vi "NI-USB6212.vi"() -> ()   [LabVIEW 2020]
uses:
  <vilib>/Utility/miscctls.llb/LVPointTypeDef.ctl
  LabVIEW 2020 Toolkits/toolkits_lv2020_32bit/Synchronization.llb/SynchRefs_SetGet.ctl
  LabVIEW 2020 Toolkits/VI Server Toolkit/VI Server Libraries/VI Server_GetControl.llb/VI Server_STR_Get.vi
  LabVIEW 2020 Toolkits/VI Server Toolkit/VI Server Libraries/VI Server_Set Controls.llb/Set STR Control.vi
  LabVIEW 2020 Toolkits/VI Server Toolkit/VI Server Libraries/VI Server_GetControl.llb/VI Server_DBL_Get.vi
  LabVIEW 2020 Toolkits/VI Server Toolkit/VI Server Libraries/VI Server_GetControl.llb/VI Server_Slide_DBL_Get.vi
  LabVIEW 2020 Toolkits/VI Server Toolkit/VI Server Libraries/VI Server_GetControl.llb/VI Server_DAQmx_Device_Get.vi
  LabVIEW 2020 Toolkits/VI Server Toolkit/VI Server Toolkit LV2013.lvlib
panel:
  in  "LastAction.AddToSecuence":bool
  in  "Help":bool
  in  "FP.Hide":bool caption="FrontPanel.Hide"
  out "System.Message":string="Instrument Initialization Successful." caption="System Message"
  in  "EXIT":bool
  in  "Tab.Main":T1(tab)
  in  "AI.Graph.Plots":u16(ring) items=["NI-USB6343/ai0", "NI-USB6343/ai1"]
  out "AI.WaveformGraph":waveform(dbl)[](graph) caption="Waveform Graph"
  in  "AI.PhysicalChannel.Include":bool
  in  "AI.MultiChannelAcquisition":bool
  out "AI.ActualSampleRate":dbl=1000.0 caption="Actual Sample Rate" format="%0.2f"
  out "AI.Averaged.Mesurement":dbl caption="Averaged Mesurement" format="%0.4f V"
  in  "AI.Measure":bool
  in  "AI.Number.Of.Samples":i32=100 caption="Number Of Samples"
  in  "AI.SampleRate":dbl=1000.0 caption="Sample Rate" format="%0.0f Hz"
  in  "AI.MinInputLimit":dbl caption="Min Input Limit" min=-10.0 max=10.0 format="%0.3f V"
  in  "AI.MaxInputLimit":dbl caption="Max Input Limit" min=-10.0 max=10.0 format="%0.3f V"
  in  "AI.TerminalConfiguration":u16(ring)=65535 caption="Terminal Configuration" items=["default"=65535, "RSE"=10083, "NRSE"=10078, "Differential"=10106, "Pseudodifferential"=12529]
  in  "AI.Sample.Mode":u16(ring)=12522 caption="Sample Mode" items=["Finite Samples"=10178, "Continuous Samples"=10123]
  in  "AI.Physical.Channel":tag="Dev1/ai0" caption="Physical Channel"
  in  "AO.Update":bool
  out "AO.WaveformGraph":waveform(dbl)(graph) caption="Waveform Graph"
  in  "AO.SampleMode":u16(ring) caption="Sample Mode" items=["Finite Samples"=10178, "Continious Samples"=10123]
  in  "AO.OutputVoltage":dbl(slide) caption="Amplitude" scale=-10.0..10.0 scale format="%0.3f V"
  in  "AO.SinewaveFrequency":dbl=10.0 caption="Sinewave Frequency" format="%0.2p Hz"
  in  "AO.GenerationMode":u16(ring) caption="Generation Mode" items=["Voltage DC", "Voltage Sine Wave Generation", "Voltage Triangle Wave Generation", "Voltage Square Wave Generation", "Voltage Sawtooth Wave Generation"]
  in  "AO.NumberOfSamples":i32=1000 caption="Number Of Samples" min=2
  in  "AO.SampleRate":dbl=1000.0 caption="Sample Rate"
  in  "AO.Sample.Clock.Source":tag="OnboardClock" caption="Sample Clock Source"
  out "AO.ActualSampleRate":dbl=1000.0 caption="Actual Sample Rate" format="%0.2f"
  in  "AO.MaxVoltage":dbl=5.0 caption="Max Voltage" format="%0.3f V"
  in  "AO.MinVoltage":dbl=-5.0 caption="Min Voltage" format="%0.3f V"
  in  "AO.Physical.Channel":tag="Dev1/ai0" caption="Physical Channel"
  in  "AO.Output":bool
  in  "DO.Port.Mask.Apply":bool
  in  "DO.Port.Lines.15:8.Mask":u8 caption="Port&Lines 15:8" format="%08b"
  in  "DO.Port.Lines.7:0.Mask":u8 caption="Port&Lines 7:0" format="%08b"
  out "DO.Port.State.Verify":bool caption="Verified"
  out "DO.Line.State.Verify":bool caption="Verified"
  in  "DO.Line.State":bool caption="State"
  in  "DO.Line":tag="Dev1/port0/line0:7" caption="Line"
  in  "DO.Line.Update":bool caption="Update:"
  in  "DO.Port.Update":bool
  in  "DO.Port.Lines.15:8":u8 caption="Port&Lines 15:8" format="%08b"
  in  "DO.Port.Lines.7:0":u8 caption="Port&Lines 7:0" format="%08b"
  in  "DO.Port":tag="Dev1/port0/line0:7" caption="Port"
  out "DI.Line.State":bool caption="State"
  in  "DI.Port.Update":bool
  out "DI.Port.Lines.8:15":u8 caption="Port&Lines 15:8" format="%08b"
  out "DI.Port.Lines.0:7":u8 caption="Port&Lines 7:0" format="%08b"
  in  "DI.Port":tag="Dev1/port0/line0:7" caption="Port"
  in  "DI.Line":tag="Dev1/port0/line0:7" caption="Line"
  in  "DI.Line.Update":bool caption="Update:"
  out "ctr1.Out.Duty Cycle.Actual":dbl caption="Ctr1: Duty Cycle Actual" format="%.2f"
  out "ctr1.Out.Frequency.Actual":dbl caption="Ctr1: Frequency Actual" format="%0.3f Hz"
  out "ctr0.Out.Duty Cycle.Actual":dbl caption="Ctr0: Duty Cycle Actual" format="%.2f"
  out "ctr0.Out.Frequency.Actual":dbl caption="Ctr0: Frequency Actual" format="%0.3f Hz"
  in  "Cntr.Out.NumberOfPulces":i32=1000 caption="Number Of Pulces" min=1
  in  "Cntr.Out.Start":bool
  in  "Cntr.Out.Sample.Mode":u16(ring)=10123 caption="Sample Mode" items=["Finite Samples"=10178, "Continuous Samples"=10123, "Hardware Timed Single Point"=12522]
  in  "Cntr.Out.Duty.Cycle":dbl=0.5 caption="Duty Cycle" format="%.2f %"
  in  "Cntr.Out.Frequency":dbl=1.0 caption="Frequency" format="%0.3f Hz"
  in  "Cntr.Out.Output.Terminal":tag="/Dev1/PFI12" caption="Output Terminal"
  in  "Cntr.Out.Channel":tag="Dev1/ctr0" caption="Channel"
  out "ctr1.In.Count":u32 caption="Count.1:"
  out "ctr0.In.Count":u32 caption="Count.0:"
  in  "Cntr.In.Start":bool
  in  "Cntr.In.IntegrationTime":u32=10 format="%.0f msec"
  in  "Cntr.In.Sample.Clock.Source":tag="PFI0" caption="Sample Clock Source"
  in  "Cntr.In.ActiveEdge":u16(ring)=10280 caption="Active Edge" items=["Rising"=10280, "Falling"=10171]
  in  "Cntr.In.Input.Terminal":tag="PFI8" caption="Input.Terminal"
  in  "Cntr.In.Channel":tag="Dev1/port0/line0:7" caption="Channel Name"
  in  "TestCase.Execute.Step.Pause":bool
  in  "TestCase.Execute.Steps":u16(ring) caption="Test Case: Pause Before Step" items=["1", "2", "3", "4", "5", "6", "7", "8", "9", "10"]
  in  "TestCase.Execute.ABORT":bool
  in  "TestCase.Execute.Next":bool
  in  "TestCase.Execute.Pause":bool
  out "TestCase.ExecutionTime":dbl caption="Execution Time:" format="%0.3f sec"
  in  "TestCase.Execution.StepTime":u32 caption="Seq. Execution: Step Time" format="%d msec"
  in  "TestCase.Execute.All":bool
  in  "TestCase.Execute.Selected":bool
  out "TestCase.SAVE.Success":bool
  in  "TestCase.SAVE":bool
  in  "SequenceFile.Open":bool
  in  "SequenceFile":path caption="Secuence File"
  in  "TestCaseConfiguration":i32[](listbox) caption="Test Case Configuration"
  in  "TestCase.StepDescription":string caption="Step Description:"
  in  "ProductType":string="USB-6343 (BNC)" caption="Product Type"
  in  "VI.WindowsTitle":string caption="Windows Title"
  in  "DAQmx.Device":tag caption="DAQmx: Device"
  in  "Cont.Measurements.CycleTime":u32 caption="Continius Measurements:\nCycleTime"
  in  "UDP.Test.String2.Send":bool
  in  "UDP.Test.String2":string caption="UDP: Test String 2"
  in  "UDP.Port.BC":u16=58433 caption="UDP: Port.BC"
  in  "UDP.Port.RT":u16=58432 caption="UDP: Port.RT"
  in  "UDP.LocalPort.Write":u16=58434 caption="UDP: Local Port.Write"
  in  "UDP.IP.Address":string="234.5.6.7" caption="UDP: IP Address"
  in  "UDP.Test.String1.Send":bool
  in  "UDP.Test.String1":string caption="UDP: Test String 1"
  in  "UDP.Responce.String.Monitor":bool
  out "UDP.ExecEng.Message.String":string caption="UDP: Execution Engine Message String"
  out "error out":errorcluster={"status"=TRUE, "code"=1055, "source"="Property Node in VI Server Toolkit LV2013.lvlib:VI server_Set Control Value from String Format.vi:5200001->DMM6500_UDP_ExecEng_Instruction_APPLY.vi->DMM6500_UDP_MAIN.vi->Keithley2100.vi"}
  in  "error in":errorcluster
  # "Important Note: Analog Input configuration shall\nstart from Physical Channel selection!"
  # "Digital Output Port\nMASK"
  # "Instructions:\n1: Active Bit; 0: Masked Bit"
  # "Digital Output"
  # "Digital Input"
  # "Counter Output"
  # "Counter Input"
  # "Counter Input"
  # "M"
  # "Multicast IP addresses must be in the 224.0.0.0 to 239.255.255.255 range."
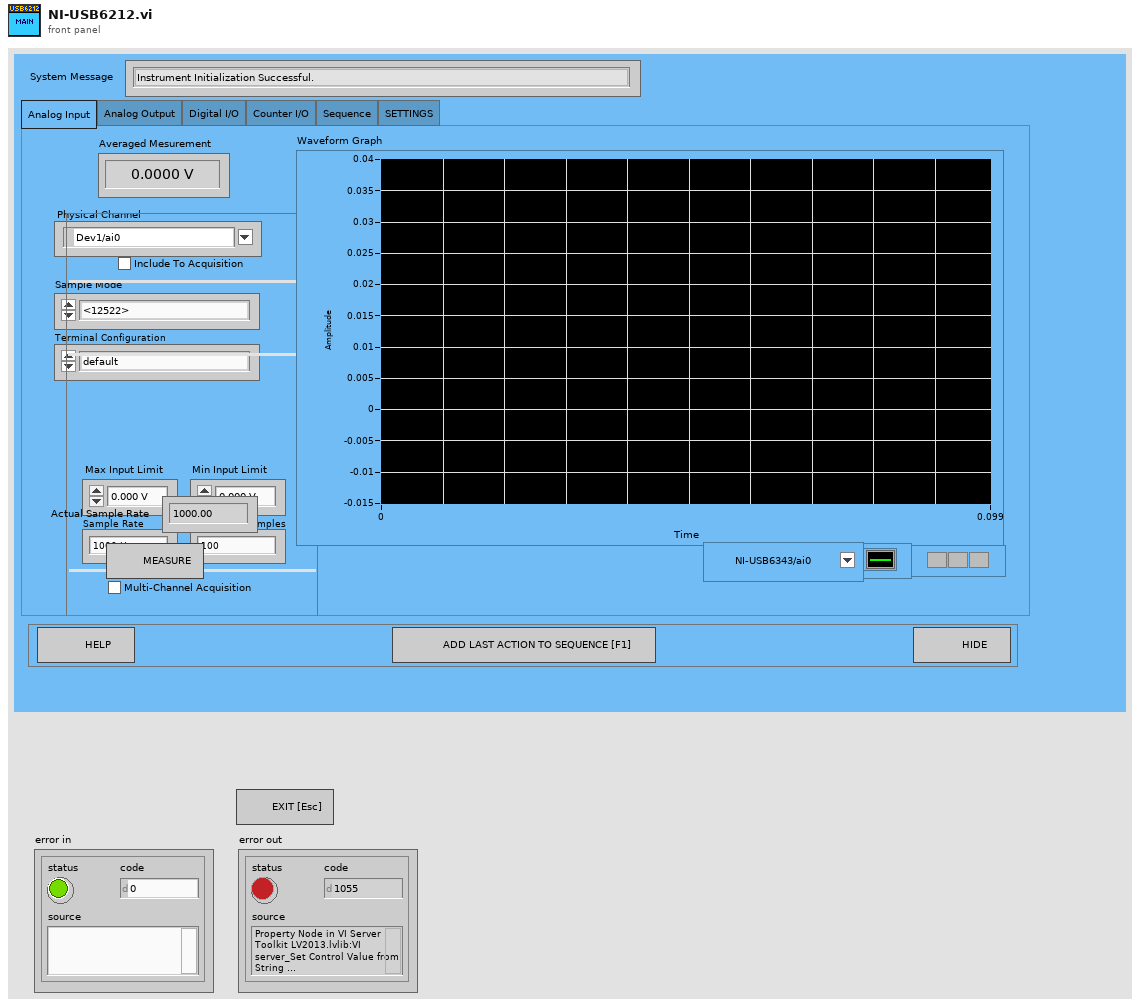
[diagram p1: front panel]
types:
  T1 = enum32{"Analog Input", "Analog Output", "Digital I/O", "Counter I/O", "Sequence", "SETTINGS"}
  T2 = typedef "LVPointTypeDef.ctl" = cluster{"Horizontal":i16, "Vertical":i16}
  T3 = typedef "VI Server_RefsCluster.ctl" = cluster{"Labels":string[], "Refs":refnum<vi>[], "VI Ref":refnum<vi>}
  T4 = typedef "SynchRefs_SetGet.ctl" = enum16{"Set", "Get"}
  T5 = enum8{"Enabled", "Disabled", "Disabled and Grayed Out"}
  T6 = cluster{"Color":u32, "PointStyle":u8, "LineStyle":u8, "Interp":u8, "LineWidth":u8, "BarPlotStyle":u8, "FillTo":i16, "XScaleIdx":u32, "YScaleIdx":u32, "Anti-Aliased":bool, "LabelFormat":u8, "TransitionType":u8, "TransitionLocation":u8, "DigitalLineStyle":u8}
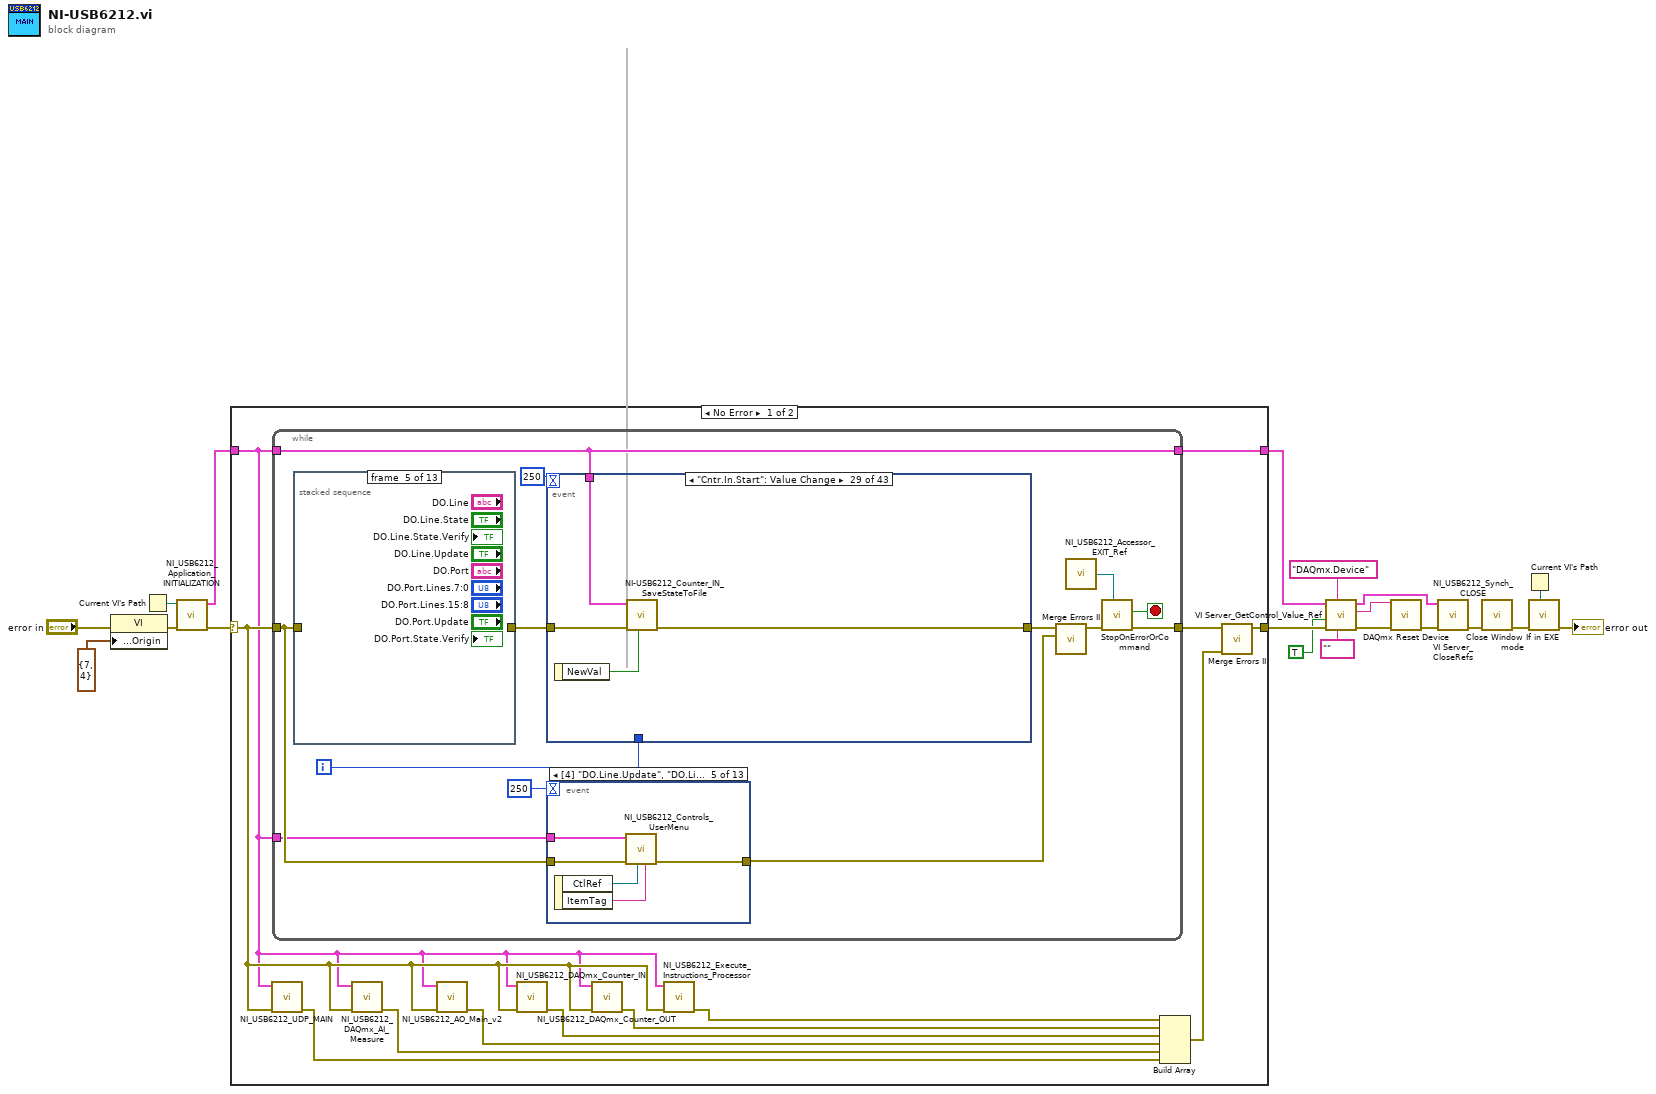
[diagram p0: block diagram]
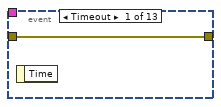
[diagram p2: hidden frame]
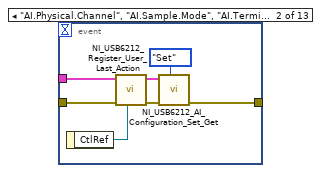
[diagram p3: hidden frame]
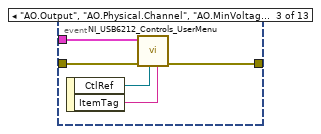
[diagram p4: hidden frame]
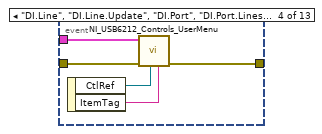
[diagram p5: hidden frame]
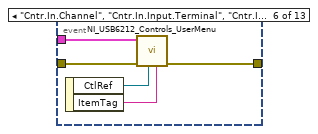
[diagram p6: hidden frame]
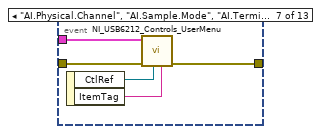
[diagram p7: hidden frame]
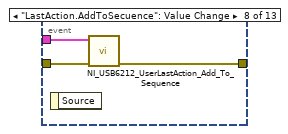
[diagram p8: hidden frame]
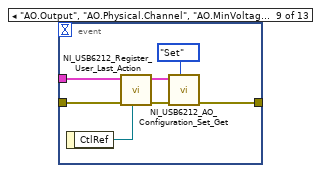
[diagram p9: hidden frame]
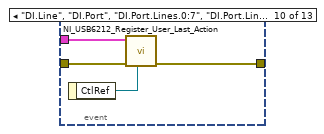
[diagram p10: hidden frame]
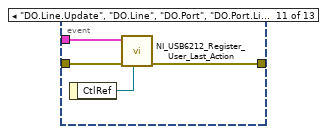
[diagram p11: hidden frame]
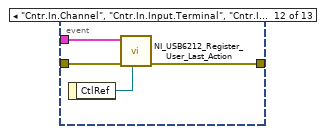
[diagram p12: hidden frame]
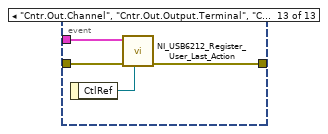
[diagram p13: hidden frame]
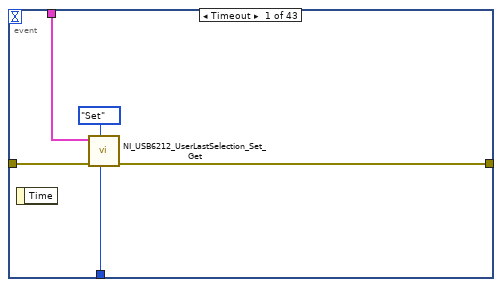
[diagram p14: hidden frame]
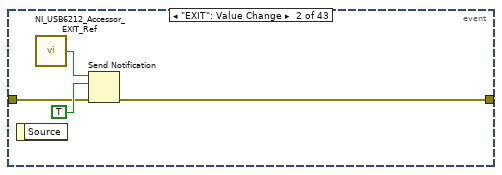
[diagram p15: hidden frame]
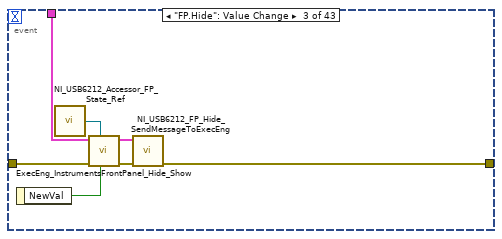
[diagram p16: hidden frame]
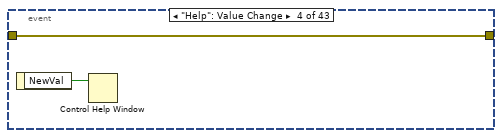
[diagram p17: hidden frame]
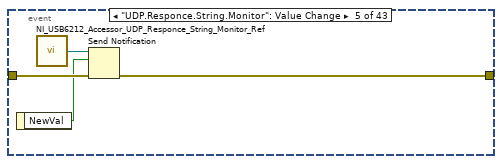
[diagram p18: hidden frame]
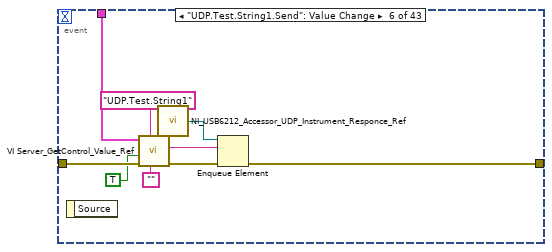
[diagram p19: hidden frame]
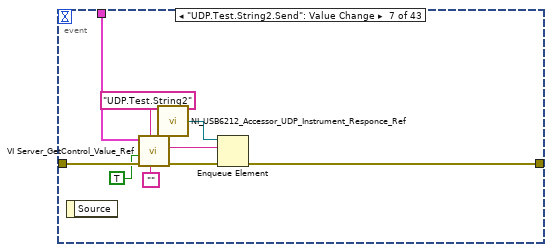
[diagram p20: hidden frame]
diagram:
  n1 = property class="VI"(error in="error in", "Front Panel Window:Origin"=T2 {"Horizontal"=7, "Vertical"=4}) -> (error out=w1:errorcluster)  [unwired: 1 in, 1 out]
  n2 = Current VI's Path() -> (path=w2:path)
  n3 = call "NI_USB6212_Application_INITIALIZATION.vi"("error in (no error)"=w1, "Top VI Path"=w2) -> ("error out"=w18:errorcluster, "VI Server Cluster DUP"=w17:T3)  [unwired: 8 in]
  n4 = case shown="No Error" w18 {
    selector: w18 -> [w22 w341]
    tunnel: [w28 w341] -> w10
    tunnel: w17 -> [w21 w340]
    tunnel: [w31 w340] -> w7
    frame No Error {
      n5 = call "NI_USB6212_UDP_MAIN.vi"("error in (no error)"=w22, "VI Server.RefsCluster"=w21) -> ("error out"=w30:errorcluster)  [unwired: 9 in]
      n6 = while {
        tunnel: w22 -> [w36]
        tunnel: [w40] -> w29
        tunnel: w21 -> [w41]
        tunnel: [w41] -> w31
        tunnel: w21 -> [w35]
        i -> [w42]
        stop <- w39 stop-if-true
        n7 = stacked-sequence {
          tunnel: w36 -> [w339 _ _ _ _ _ _ _ _ _ _ _ _]
          tunnel: [w339 _ _ _ _ _ _ _ _ _ _ _ _] -> w44
          frame #0 {
          }
          frame #1 {
          }
          frame #2 {
          }
          frame #3 {
          }
          frame #4 {
          }
          frame #5 {
          }
          frame #6 {
          }
          frame #7 {
          }
          frame #8 {
          }
          frame #9 {
          }
          frame #10 {
          }
          frame #11 {
          }
          frame #12 {
          }
        }
        n8 = event shown="[28] \"Cntr.In.Start\": Value Change" {
          selector: _ -> [_ _ _ _ _ _ _ _ _ _ _ _ _ _ _ _ _ _ _ _ _ _ _ _ _ _ _ _ _ _ _ _ _ _ _ _ _ _ _ _ _ _ _]
          dyn-events: _ -> [_ _ _ _ _ _ _ _ _ _ _ _ _ _ _ _ _ _ _ _ _ _ _ _ _ _ _ _ _ _ _ _ _ _ _ _ _ _ _ _ _ _ _]
          timeout: 250 -> [_ _ _ _ _ _ _ _ _ _ _ _ _ _ _ _ _ _ _ _ _ _ _ _ _ _ _ _ _ _ _ _ _ _ _ _ _ _ _ _ _ _ _]
          tunnel: w44 -> [w107 w109 w118 w121 w125 w134 w143 w147 w160 w164 w169 w170 w173 w180 w184 w188 w194 w202 w227 w230 w234 w237 w240 w244 w247 w250 w259 w267 w270 w274 w285 w291 w294 w306 w309 w313 w316 w319 w322 w326 w330 w334 w338]
          tunnel: w42 -> [w106 _ _ _ _ _ _ _ _ _ _ _ _ _ _ _ _ _ _ _ _ _ _ _ _ _ _ _ _ _ _ _ _ _ _ _ _ _ _ _ _ _ _]
          tunnel: [w104 w111 w119 w121 w123 w132 w141 w145 w157 w161 w165 w170 w172 w176 w181 w187 w193 w196 w215 w229 w232 w235 w238 w243 w245 w248 w256 w265 w271 w272 w279 w290 w293 w304 w307 w311 w314 w318 w321 w324 w329 w333 w337] -> w34
          tunnel: w41 -> [w105 _ w115 _ _ w131 w140 w144 w159 w163 w168 _ w171 w179 w183 _ _ w201 w225 w228 w233 w236 w239 w242 w246 w249 _ w266 w269 w273 w284 w289 w292 w305 w308 w312 w315 w317 w320 _ _ _ _]
          event Timeout {
            n9 = event-data() -> ()  [unwired: 1 in, 1 out]
            n10 = call "NI_USB6212_UserLastSelection_Set_Get.vi"("LoopCounter"=w106, "SynchRefs.Set/Get"=SynchRefs_SetGet."Set", "error in"=w107, "VI Server.RefsCluster"=w105) -> ("error out"=w104:errorcluster)  [unwired: 6 in, 1 out]
          }
          event "EXIT": Value Change {
            n11 = event-data() -> ()  [unwired: 1 in, 1 out]
            n12 = call "NI_USB6212_Accessor_EXIT_Ref.vi"() -> ("EXIT"=w112:refnum<notifier>)  [unwired: 6 in]
            n13 = Send Notification(notification=TRUE, notifier=w112, error in (no error)=w109) -> (error out=w111:errorcluster)  [unwired: 1 out]
          }
          event "FP.Hide": Value Change {
            n14 = event-data() -> ("NewVal"=w116:bool)  [unwired: 1 in]
            n15 = call "NI_USB6212_Accessor_FP_State_Ref.vi"() -> ("FP.State"=w113:refnum<notifier>)  [unwired: 6 in]
            n16 = call "ExecEng_InstrumentsFrontPanel_Hide_Show.vi"("FP.Hide/Show"=w116, "FP.State"=w113, "error in (no error)"=w118, "VI Server Cluster"=w115) -> ("error out"=w117:errorcluster, "VI Server Cluster DUP"=w114:T3)  [unwired: 6 in]
            n17 = call "NI_USB6212_FP_Hide_SendMessageToExecEng.vi"("error in (no error)"=w117, "VI Server Cluster"=w114) -> ("error out"=w119:errorcluster)  [unwired: 9 in]
          }
          event "Help": Value Change {
            n18 = event-data() -> ("NewVal"=w120:bool)  [unwired: 1 in]
            n19 = Control Help Window(1:w120) -> ()  [unwired: 1 in]
          }
          event "UDP.Responce.String.Monitor": Value Change {
            n20 = event-data() -> ("NewVal"=w122:bool)  [unwired: 1 in]
            n21 = call "NI_USB6212_Accessor_UDP_Responce_String_Monitor_Ref.vi"() -> ("UDP.ExecEng.Command.String.Monitor"=w124:refnum<notifier>)  [unwired: 6 in]
            n22 = Send Notification(notification=w122, notifier=w124, error in (no error)=w125) -> (error out=w123:errorcluster)  [unwired: 1 out]
          }
          event "UDP.Test.String1.Send": Value Change {
            n23 = event-data() -> ()  [unwired: 1 in, 1 out]
            n24 = call-poly "VI Server_GetControl_Value_Ref.vi"("DataType"="", "Control.Label"="UDP.Test.String1", "error in"=w134, "SingleInstance"=TRUE, "VI Server.RefsCluster"=w131) -> ("error out"=w133:errorcluster, "Value"=w126:string)  [unwired: 3 in, 2 out]
            n25 = call "NI_USB6212_Accessor_UDP_Instrument_Responce_Ref.vi"() -> ("UDP.Instrument.Responce.Q"=w127:refnum<queue>)  [unwired: 6 in]
            n26 = Enqueue Element(queue=w127, element=w126, error in (no error)=w133) -> (error out=w132:errorcluster)  [unwired: 1 in, 2 out]
          }
          event "UDP.Test.String2.Send": Value Change {
            n27 = event-data() -> ()  [unwired: 1 in, 1 out]
            n28 = call-poly "VI Server_GetControl_Value_Ref.vi"("DataType"="", "Control.Label"="UDP.Test.String2", "error in"=w143, "SingleInstance"=TRUE, "VI Server.RefsCluster"=w140) -> ("error out"=w142:errorcluster, "Value"=w135:string)  [unwired: 3 in, 2 out]
            n29 = call "NI_USB6212_Accessor_UDP_Instrument_Responce_Ref.vi"() -> ("UDP.Instrument.Responce.Q"=w136:refnum<queue>)  [unwired: 6 in]
            n30 = Enqueue Element(queue=w136, element=w135, error in (no error)=w142) -> (error out=w141:errorcluster)  [unwired: 1 in, 2 out]
          }
          event "UDP.ExecEng.Message.String": Shortcut Menu Selection (User) {
            n31 = event-data() -> ("ItemTag"=w146:string)  [unwired: 1 in]
            n32 = case shown="\"Clear Indicator\"" w146 {
              tunnel: w147 -> [w148 w154]
              tunnel: [w148 w153] -> w145
              tunnel: w144 -> [_ w152]
              frame "", Default {
              }
              frame "Clear Indicator" {
                n33 = call-poly "VI Server_Set Control Value.vi"("New Value"="", "Label"="UDP.ExecEng.Message.String" ("Control.Label"), "error in"=w154, "Single Instance (T)"=TRUE ("SingleInstance"), "VI Server Cluster"=w152) -> ("error out"=w153:errorcluster)  [unwired: 4 in, 2 out]
              }
            }
          }
          event "DAQmx.Device": Value Change {
            n34 = event-data() -> ("NewVal"=w156:tag)  [unwired: 1 in]
            n35 = call "NI_USB6212_DAQmx_LimitPhysicalChannelsToDevice.vi"("error in (no error)"=w160, "VI Server Cluster"=w159) -> ("error out"=w158:errorcluster, "VI Server Cluster.DUP"=w155:T3)  [unwired: 7 in, 1 out]
            n36 = call "NI_USB6212_DAQmx_DeviceName_Changed_UpdateSet_Get_Sections.vi"("DAQmx.Device"=w156, "error in (no error)"=w158, "VI Server Cluster"=w155) -> ("error out"=w157:errorcluster)  [unwired: 8 in]
          }
          event "AI.Physical.Channel": Value Change {
            n37 = event-data() -> ()  [unwired: 1 in, 1 out]
            n38 = call "NI_USB6212_AI_Configuration_Set_Get.vi"("SynchRefs.Set/Get"=SynchRefs_SetGet."Get", "error in (no error)"=w164, "VI Server Cluster"=w163) -> ("error out"=w161:errorcluster)  [unwired: 6 in, 2 out]
          }
          event "AI.WaveformGraph": Plot Attribute Change {
            n39 = event-data() -> ("OldAttrib"=w167:T6, "NewAttrib"=w166:T6)  [unwired: 1 in]
            n40 = call "NI_USB6212_AI_Graph_PlotAttribute_ValueChanged.vi"("NewAttrib"=w166, "OldAttrib"=w167, "error in (no error)"=w169, "VI Server Cluster"=w168) -> ("error out"=w165:errorcluster)  [unwired: 7 in]
          }
          event "AI.Measure": Value Change {
            n41 = event-data() -> ()  [unwired: 1 in, 1 out]
          }
          event "AO.Physical.Channel": Value Change {
            n42 = event-data() -> ()  [unwired: 1 in, 1 out]
            n43 = call "NI_USB6212_AO_Configuration_Set_Get.vi"("error in (no error)"=w173, "VI Server Cluster"=w171) -> ("error out"=w172:errorcluster)  [unwired: 7 in, 2 out]
          }
          event "AO.GenerationMode": Value Change {
            n44 = event-data() -> ("NewVal"=w174:u16)  [unwired: 1 in]
            n45 = call "NI_USB6212_AO_GenerationMode.vi"("AO.GenerationMode"=w174, "error in (no error)"=w180, "VI Server Cluster"=w179) -> ("error out"=w177:errorcluster)  [unwired: 7 in, 1 out]
            n46 = call "NI_USB6212_Accessor_ao_Waveform_Array_Update_Ref.vi"() -> ("ao.Waveform.Array.Update"=w175:refnum<notifier>)  [unwired: 6 in]
            n47 = Send Notification(notification=TRUE, notifier=w175, error in (no error)=w177) -> (error out=w176:errorcluster)  [unwired: 1 out]
          }
          event "AO.OutputVoltage", "AO.SinewaveFrequency": Value Change {
            n48 = event-data() -> ()  [unwired: 1 in, 1 out]
            n49 = call "VI Server_CycleEventBySignalingValue.vi"("Label"="AO.GenerationMode", "error in"=w184, "VI Server.RefsCluster"=w183) -> ("error out"=w181:errorcluster)  [unwired: 7 in, 1 out]
          }
          event "AO.Output": Value Change {
            n50 = event-data() -> ("NewVal"=w186:bool)  [unwired: 1 in]
            n51 = call "NI_USB6212_Accessor_ao0_State_Ref.vi"() -> ("ao0.State"=w189:refnum<notifier>)  [unwired: 6 in]
            n52 = Send Notification(notification=w186, notifier=w189, error in (no error)=w188) -> (error out=w191:errorcluster)  [unwired: 1 out]
            n53 = call "NI_USB6212_Accessor_ao_Waveform_Array_Update_Ref.vi"() -> ("ao.Waveform.Array.Update"=w190:refnum<notifier>)  [unwired: 6 in]
            n54 = Send Notification(notification=TRUE, notifier=w190, error in (no error)=w191) -> (error out=w187:errorcluster)  [unwired: 1 out]
          }
          event "AO.Update": Value Change {
            n55 = event-data() -> ()  [unwired: 1 in, 1 out]
            n56 = call "NI_USB6212_Accessor_ao_Waveform_Array_Update_Ref.vi"() -> ("ao.Waveform.Array.Update"=w195:refnum<notifier>)  [unwired: 6 in]
            n57 = Send Notification(notification=TRUE, notifier=w195, error in (no error)=w194) -> (error out=w193:errorcluster)  [unwired: 1 out]
          }
          event "AO.Sample.Clock.Source", "AO.SampleMode", "AO.SampleRate", "AO.NumberOfSamples": Value Change {
            n58 = event-data() -> ()  [unwired: 1 in, 1 out]
            n59 = call "NI_USB6212_Accessor_ao0_State_Ref.vi"() -> ("ao0.State"=w199:refnum<notifier>)  [unwired: 6 in]
            n60 = call "NI_USB6212_AO_ConfigurationAtributes.vi"("error in (no error)"=w202, "VI Server Cluster"=w201) -> ("error out"=w197:errorcluster)  [unwired: 8 in, 1 out]
            n61 = Get Notifier Status(notifier=w199, error in (no error)=w197) -> (current notification=w200:bool, error out=w198:errorcluster)  [unwired: 3 out]
            n62 = case shown="True" w200 {
              tunnel: [w203 w208] -> w196
              tunnel: w198 -> [w203 w205]
              tunnel: w199 -> [_ w204]
              frame False {
              }
              frame True {
                w207 = TRUE ("notification")
                n63 = Send Notification(notification=FALSE, notifier=w204, error in (no error)=w205) -> (error out=w210:errorcluster)  [unwired: 1 out]
                n64 = call "NI_USB6212_Accessor_ao_Waveform_Array_Update_Ref.vi"() -> ("ao.Waveform.Array.Update"=w211:refnum<notifier>)  [unwired: 6 in]
                n65 = Send Notification(notification=w207, notifier=w211, error in (no error)=w210) -> (error out=w209:errorcluster)  [unwired: 1 out]
                n66 = Send Notification(notification=w207, notifier=w204, error in (no error)=w209) -> (error out=w208:errorcluster)  [unwired: 1 out]
              }
            }
          }
          event "AO.MaxVoltage", "AO.MinVoltage": Value Change {
            w218 = 0.0
            w217 = TRUE ("SingleInstance")
            n67 = event-data() -> ()  [unwired: 1 in, 1 out]
            n68 = call-poly "VI Server_GetControl_Value_Ref.vi"("DataType"=w218, "Control.Label"="AO.MaxVoltage", "error in"=w227, "SingleInstance"=w217, "VI Server.RefsCluster"=w225) -> ("error out"=w226:errorcluster, "Value"=w212:dbl, "VI Server.RefsCluster.DUP"=w224:T3)  [unwired: 3 in, 1 out]
            n69 = call-poly "VI Server_GetControl_Value_Ref.vi"("DataType"=w218, "Control.Label"="AO.MinVoltage", "error in"=w226, "SingleInstance"=w217, "VI Server.RefsCluster"=w224) -> ("error out"=w221:errorcluster, "Value"=w213:dbl, "VI Server.RefsCluster.DUP"=w220:T3)  [unwired: 3 in, 1 out]
            n70 = call-poly "VI Server_GetControl_Value_Ref.vi"("DataType"=w218, "Control.Label"="AO.OutputVoltage", "error in"=w221, "SingleInstance"=w217, "VI Server.RefsCluster"=w220) -> ("error out"=w216:errorcluster, "Control.Ref"=w214:refnum<vi>)  [unwired: 3 in, 2 out]
            n71 = property class="Slide (strict)"(reference=w214, error in=w216, "Scale.Minimum"=w213, "Scale.Maximum"=w212) -> (error out=w215:errorcluster)  [unwired: 1 out]
          }
          event "DI.Line.Update": Value Change {
            n72 = event-data() -> ()  [unwired: 1 in, 1 out]
            n73 = call "NI_USB6212_Digital_Input_Line_Update.vi"("error in (no error)"=w230, "VI Server Cluster"=w228) -> ("error out"=w229:errorcluster)  [unwired: 9 in]
          }
          event "DI.Port": Value Change {
            n74 = event-data() -> ("NewVal"=w231:tag)  [unwired: 1 in]
            n75 = call "NI_USB6212_DI_Port_ValueChanged.vi"("DI.Port"=w231, "error in (no error)"=w234, "VI Server Cluster"=w233) -> ("error out"=w232:errorcluster)  [unwired: 8 in]
          }
          event "DI.Port.Update": Value Change {
            n76 = event-data() -> ()  [unwired: 1 in, 1 out]
            n77 = call "NI_USB6212_DI_Port_Update.vi"("error in (no error)"=w237, "VI Server Cluster"=w236) -> ("error out"=w235:errorcluster)  [unwired: 9 in]
          }
          event "DO.Line.Update": Value Change {
            n78 = event-data() -> ()  [unwired: 1 in, 1 out]
            n79 = call "NI_USB6212_Digital_Output_Line_Update.vi"("error in (no error)"=w240, "VI Server Cluster"=w239) -> ("error out"=w238:errorcluster)  [unwired: 9 in]
          }
          event "DO.Port": Value Change {
            n80 = event-data() -> ("NewVal"=w241:tag)  [unwired: 1 in]
            n81 = call "NI_USB6212_DO_Port_ValueChanged.vi"("DO.Port"=w241, "error in (no error)"=w244, "VI Server Cluster"=w242) -> ("error out"=w243:errorcluster)  [unwired: 8 in]
          }
          event "DO.Port.Update": Value Change {
            n82 = event-data() -> ()  [unwired: 1 in, 1 out]
            n83 = call "NI_USB6212_DO_Port_Update.vi"("error in (no error)"=w247, "VI Server Cluster"=w246) -> ("error out"=w245:errorcluster)  [unwired: 9 in]
          }
          event "DO.Port.Mask.Apply": Value Change {
            n84 = event-data() -> ()  [unwired: 1 in, 1 out]
            n85 = call "NI_USB6212_DO_Port_Mask_Apply.vi"("error in (no error)"=w250, "VI Server Cluster"=w249) -> ("error out"=w248:errorcluster)  [unwired: 9 in]
          }
          event "DO.Port.Lines.7:0", "DO.Port.Lines.15:8", "DI.Port.Lines.0:7", "DI.Port.Lines.8:15", "DO.Port.Lines.7:0.Mask", "DO.Port.Lines.15:8.Mask": Mouse Down {
            n86 = event-data() -> ("CtlRef"=w258:refnum<vi>)  [unwired: 1 in]
            n87 = property class="DigNum (strict)"(reference=w258, error in=w259) -> (reference out=w255:refnum<vi>, error out=w257:errorcluster, "FormatString"=w252:string)
            n88 = Match Pattern(string=w252, regular expression="[0-9]+") -> (after substring=w251:string)  [unwired: 1 in, 3 out]
            n89 = case shown="\"b\", Default" w251 {
              tunnel: ["%.0f" "%02x" "%02o" "%08b"] -> w254
              frame "f" {
              }
              frame "x" {
              }
              frame "o" {
              }
              frame "b", Default {
              }
            }
            n90 = property class="DigNum (strict)"(reference=w255, error in=w257, "FormatString"=w254) -> (error out=w256:errorcluster)  [unwired: 1 out]
          }
          event "Cntr.In.Channel": Value Change {
            n91 = event-data() -> ("NewVal"=w264:tag)  [unwired: 1 in]
            n92 = call "NI-USB6212_Counter_IN_GetStateFromFile.vi"("Counter.IN.Channel"=w264, "error in (no error)"=w267, "VI Server Cluster"=w266) -> ("error out"=w265:errorcluster)  [unwired: 7 in, 1 out]
          }
          event "Cntr.In.Start": Value Change {
            n93 = event-data() -> ("NewVal"=w268:bool)  [unwired: 1 in]
            n94 = call "NI-USB6212_Counter_IN_SaveStateToFile.vi"("Cntr.In.Start"=w268, "error in (no error)"=w270, "VI Server Cluster"=w269) -> ("error out"=w271:errorcluster)  [unwired: 7 in, 1 out]
          }
          event "Cntr.Out.Channel": Value Change {
            n95 = event-data() -> ("NewVal"=w275:tag)  [unwired: 1 in]
            n96 = call "NI-USB6212_Counter_OUT_GetStateFromFile.vi"("Counter.OUT.Channel"=w275, "error in (no error)"=w274, "VI Server Cluster"=w273) -> ("error out"=w272:errorcluster)  [unwired: 7 in, 1 out]
          }
          event "Cntr.Out.Sample.Mode": Value Change {
            n97 = event-data() -> ()  [unwired: 1 in, 1 out]
            n98 = call "VI Server_Get Text Ring Selection.vi"("Label"="Cntr.Out.Sample.Mode", "error in"=w285, "Single Instance (T)"=TRUE, "VI Server Cluster"=w284) -> ("error out"=w280:errorcluster, "Selection"=w281:string, "VI Server Custer.DUP"=w278:T3)  [unwired: 2 in, 3 out]
            n99 = case shown="\"Finite Samples\"" w281 {
              tunnel: [T5."Disabled and Grayed Out" ("Disabled") T5."Enabled" ("Disabled")] -> w277
              frame "Continuous Samples", Default {
              }
              frame "Finite Samples" {
              }
            }
            n100 = call "VI Server_Enable_Disable.vi"("Disabled"=w277, "Label"="Cntr.Out.NumberOfPulces", "error in"=w280, "VI Server Cluster"=w278) -> ("error out"=w279:errorcluster)  [unwired: 5 in, 2 out]
          }
          event "Cntr.Out.Start": Value Change {
            n101 = event-data() -> ("NewVal"=w288:bool)  [unwired: 1 in]
            n102 = call "NI-USB6212_Counter_OUT_SaveStateToFile.vi"("Cntr.In.Start"=w288, "error in (no error)"=w291, "VI Server Cluster"=w289) -> ("error out"=w290:errorcluster)  [unwired: 7 in, 1 out]
          }
          event "LastAction.AddToSecuence": Value Change {
            w303 = "TestCaseConfiguration" ("Label")
            w302 = TRUE ("SingleInstance")
            n103 = event-data() -> ()  [unwired: 1 in, 1 out]
            n104 = call "NI_USB6212_Accessor_RegisteredUserEvent_Ref.vi"() -> ("RegisteredUserEvent"=w295:refnum<notifier>)  [unwired: 6 in]
            n105 = Get Notifier Status(notifier=w295, error in (no error)=w294) -> (current notification=w298:string[], error out=w296:errorcluster)  [unwired: 3 out]
            n106 = call "VI Server_M_ClmnListBox_1orMoreSelection_ItemNames_GET.vi"("Label"=w303, "error in"=w296, "SingleInstance"=w302, "VI Server.RefsCluster"=w292) -> ("error out"=w299:errorcluster, "Item Names"=w297:string[][], "VI Server.RefsCluster.DUP"=w300:T3)  [unwired: 1 in, 4 out]
            n107 = Build Array (concatenate)(w297, w298) -> (w301:string[][])
            n108 = call "VI Server_M_ClmnListBox_ItemNames_SET.vi"("Item Names"=w301, "Label"=w303, "error in"=w299, "SingleInstance"=w302, "VI Server.RefsCluster"=w300) -> ("error out"=w293:errorcluster)  [unwired: 4 in, 2 out]
          }
          event "TestCase.SAVE": Value Change {
            n109 = event-data() -> ()  [unwired: 1 in, 1 out]
            n110 = call "NI_USB6212_Sequence_Save.vi"("error in (no error)"=w306, "VI Server Cluster"=w305) -> ("error out"=w304:errorcluster)  [unwired: 9 in]
          }
          event "SequenceFile.Open": Value Change {
            n111 = event-data() -> ()  [unwired: 1 in, 1 out]
            n112 = call "NI_USB6212_Sequence_Open.vi"("error in (no error)"=w309, "VI Server Cluster"=w308) -> ("error out"=w307:errorcluster)  [unwired: 9 in]
          }
          event "TestCaseConfiguration": Shortcut Menu Selection (User) {
            n113 = event-data() -> ("ItemTag"=w310:string)  [unwired: 1 in]
            n114 = call "NI_USB6212_Sequence_TestCaseConfig_UserMenu.vi"("ItemTag"=w310, "error in (no error)"=w313, "VI Server.RefsCluster"=w312) -> ("error out"=w311:errorcluster)  [unwired: 8 in]
          }
          event "TestCaseConfiguration": Value Change {
            n115 = event-data() -> ()  [unwired: 1 in, 1 out]
            n116 = call "NI_USB6212_TestCase_Configuration_ValueChanged.vi"("error in"=w316, "VI Server.RefsCluster"=w315) -> ("error out"=w314:errorcluster)  [unwired: 8 in, 1 out]
          }
          event "TestCase.Execute.Selected": Value Change {
            n117 = event-data() -> ()  [unwired: 1 in, 1 out]
            n118 = call "NI_USB6212_ExecuteSelectedInstruction.vi"("error in (no error)"=w319, "VI Server Cluster"=w317) -> ("error out"=w318:errorcluster)  [unwired: 9 in]
          }
          event "TestCase.Execute.All": Value Change {
            n119 = event-data() -> ()  [unwired: 1 in, 1 out]
            n120 = call "NI_USB6212_Execute_All_Instruction.vi"("error in (no error)"=w322, "VI Server Cluster"=w320) -> ("error out"=w321:errorcluster)  [unwired: 9 in]
          }
          event "TestCase.Execute.Pause": Value Change {
            n121 = event-data() -> ("NewVal"=w325:bool)  [unwired: 1 in]
            n122 = call "NI_USB6212_TestCase_Execution_Pause_Ref.vi"() -> ("SequenceExecution.StepPAUSE"=w323:refnum<notifier>)  [unwired: 6 in]
            n123 = Send Notification(notification=w325, notifier=w323, error in (no error)=w326) -> (error out=w324:errorcluster)  [unwired: 1 out]
          }
          event "TestCase.Execute.Next": Value Change {
            n124 = event-data() -> ()  [unwired: 1 in, 1 out]
            n125 = call "NI_USB6212_Accessor_Sequence_Execution_NEXT_Ref.vi"() -> ("SequenceExecution.NEXT"=w328:refnum<notifier>)  [unwired: 6 in]
            n126 = Send Notification(notification=TRUE, notifier=w328, error in (no error)=w330) -> (error out=w329:errorcluster)  [unwired: 1 out]
          }
          event "TestCase.Execute.ABORT": Value Change {
            n127 = event-data() -> ()  [unwired: 1 in, 1 out]
            n128 = call "NI_USB6212_Accessor_Sequence_Execution_ABORT_Ref.vi"() -> ("SequenceExecution.ABORT"=w332:refnum<notifier>)  [unwired: 6 in]
            n129 = Send Notification(notification=TRUE, notifier=w332, error in (no error)=w334) -> (error out=w333:errorcluster)  [unwired: 1 out]
          }
          event "TestCase.Execute.Step.Pause": Value Change {
            n130 = event-data() -> ("NewVal"=w336:bool)  [unwired: 1 in]
            n131 = call "NI_USB6212_TestCase_Execution_Pause_Ref.vi"() -> ("SequenceExecution.StepPAUSE"=w335:refnum<notifier>)  [unwired: 6 in]
            n132 = Send Notification(notification=w336, notifier=w335, error in (no error)=w338) -> (error out=w337:errorcluster)  [unwired: 1 out]
          }
        }
        n133 = event shown="[4] \"DO.Line.Update\", \"DO.Line\", \"DO.Port\", \"DO.Port.Lines.7:0\", \"DO.Port.Lines.15:8\", \"DO.Port.Update\", \"DO.Line.State\", \"DO.Port.Lines.7:0.Mask\", \"DO.Port.Lines.15:8.Mask\", \"DO.Port.Mask.Apply\": Shortcut Menu Selection (User)" {
          selector: _ -> [_ _ _ _ _ _ _ _ _ _ _ _ _]
          dyn-events: _ -> [_ _ _ _ _ _ _ _ _ _ _ _ _]
          timeout: 250 -> [_ _ _ _ _ _ _ _ _ _ _ _ _]
          tunnel: [w45 w46 w56 w60 w65 w70 w76 w79 w83 w89 w94 w98 w102] -> w32
          tunnel: w35 -> [_ w50 w57 w62 w67 w72 w75 w78 w86 w90 w93 w97 w101]
          tunnel: w36 -> [w45 w52 w53 w61 w66 w71 w77 w80 w87 w91 w95 w99 w103]
          event Timeout {
            n134 = event-data() -> ()  [unwired: 1 in, 1 out]
          }
          event "AI.Physical.Channel", "AI.Sample.Mode", "AI.TerminalConfiguration", "AI.MaxInputLimit", "AI.MinInputLimit", "AI.SampleRate", "AI.Number.Of.Samples", "AI.Measure", "AI.PhysicalChannel.Include", "AI.MultiChannelAcquisition": Value Change {
            n135 = event-data() -> ("CtlRef"=w51:refnum<vi>)  [unwired: 1 in]
            n136 = call "NI_USB6212_Register_User_Last_Action.vi"("CtlRef"=w51, "error in (no error)"=w52, "VI Server Cluster"=w50) -> ("error out"=w47:errorcluster, "VI Server Cluster.DUP"=w48:T3)  [unwired: 7 in]
            n137 = call "NI_USB6212_AI_Configuration_Set_Get.vi"("SynchRefs.Set/Get"=SynchRefs_SetGet."Set", "error in (no error)"=w47, "VI Server Cluster"=w48) -> ("error out"=w46:errorcluster)  [unwired: 6 in, 2 out]
          }
          event "AO.Output", "AO.Physical.Channel", "AO.MinVoltage", "AO.MaxVoltage", "AO.Sample.Clock.Source", "AO.SampleRate", "AO.NumberOfSamples", "AO.GenerationMode", "AO.SinewaveFrequency", "AO.OutputVoltage", "AO.SampleMode", "AO.Update": Shortcut Menu Selection (User) {
            n138 = event-data() -> ("CtlRef"=w55:refnum<vi>, "ItemTag"=w54:string)  [unwired: 1 in]
            n139 = call "NI_USB6212_Controls_UserMenu.vi"("ItemTag"=w54, "Control Ref"=w55, "error in (no error)"=w53, "VI Server Cluster"=w57) -> ("error out"=w56:errorcluster)  [unwired: 7 in]
          }
          event "DI.Line", "DI.Line.Update", "DI.Port", "DI.Port.Lines.0:7", "DI.Port.Lines.8:15", "DI.Port.Update": Shortcut Menu Selection (User) {
            n140 = event-data() -> ("CtlRef"=w59:refnum<vi>, "ItemTag"=w58:string)  [unwired: 1 in]
            n141 = call "NI_USB6212_Controls_UserMenu.vi"("ItemTag"=w58, "Control Ref"=w59, "error in (no error)"=w61, "VI Server Cluster"=w62) -> ("error out"=w60:errorcluster)  [unwired: 7 in]
          }
          event "DO.Line.Update", "DO.Line", "DO.Port", "DO.Port.Lines.7:0", "DO.Port.Lines.15:8", "DO.Port.Update", "DO.Line.State", "DO.Port.Lines.7:0.Mask", "DO.Port.Lines.15:8.Mask", "DO.Port.Mask.Apply": Shortcut Menu Selection (User) {
            n142 = event-data() -> ("CtlRef"=w64:refnum<vi>, "ItemTag"=w63:string)  [unwired: 1 in]
            n143 = call "NI_USB6212_Controls_UserMenu.vi"("ItemTag"=w63, "Control Ref"=w64, "error in (no error)"=w66, "VI Server Cluster"=w67) -> ("error out"=w65:errorcluster)  [unwired: 7 in]
          }
          event "Cntr.In.Channel", "Cntr.In.Input.Terminal", "Cntr.In.ActiveEdge", "Cntr.In.Sample.Clock.Source", "Cntr.In.IntegrationTime", "Cntr.In.Start", "Cntr.Out.Channel", "Cntr.Out.Output.Terminal", "Cntr.Out.Frequency", "Cntr.Out.Duty.Cycle", "Cntr.Out.Sample.Mode", "Cntr.Out.Start", "Cntr.Out.NumberOfPulces": Shortcut Menu Selection (User) {
            n144 = event-data() -> ("CtlRef"=w69:refnum<vi>, "ItemTag"=w68:string)  [unwired: 1 in]
            n145 = call "NI_USB6212_Controls_UserMenu.vi"("ItemTag"=w68, "Control Ref"=w69, "error in (no error)"=w71, "VI Server Cluster"=w72) -> ("error out"=w70:errorcluster)  [unwired: 7 in]
          }
          event "AI.Physical.Channel", "AI.Sample.Mode", "AI.TerminalConfiguration", "AI.MaxInputLimit", "AI.MinInputLimit", "AI.SampleRate", "AI.Number.Of.Samples", "AI.Measure", "AI.PhysicalChannel.Include", "AI.MultiChannelAcquisition": Shortcut Menu Selection (User) {
            n146 = event-data() -> ("CtlRef"=w74:refnum<vi>, "ItemTag"=w73:string)  [unwired: 1 in]
            n147 = call "NI_USB6212_Controls_UserMenu.vi"("ItemTag"=w73, "Control Ref"=w74, "error in (no error)"=w77, "VI Server Cluster"=w75) -> ("error out"=w76:errorcluster)  [unwired: 7 in]
          }
          event "LastAction.AddToSecuence": Value Change {
            n148 = event-data() -> ()  [unwired: 1 in, 1 out]
            n149 = call "NI_USB6212_UserLastAction_Add_To_Sequence.vi"("error in (no error)"=w80, "VI Server Cluster"=w78) -> ("error out"=w79:errorcluster)  [unwired: 9 in]
          }
          event "AO.Output", "AO.Physical.Channel", "AO.MinVoltage", "AO.MaxVoltage", "AO.Sample.Clock.Source", "AO.SampleRate", "AO.NumberOfSamples", "AO.GenerationMode", "AO.SinewaveFrequency", "AO.OutputVoltage", "AO.SampleMode", "AO.Update": Value Change {
            n150 = event-data() -> ("CtlRef"=w85:refnum<vi>)  [unwired: 1 in]
            n151 = call "NI_USB6212_Register_User_Last_Action.vi"("CtlRef"=w85, "error in (no error)"=w87, "VI Server Cluster"=w86) -> ("error out"=w84:errorcluster, "VI Server Cluster.DUP"=w82:T3)  [unwired: 7 in]
            n152 = call "NI_USB6212_AO_Configuration_Set_Get.vi"("SynchRefs.Set/Get"=SynchRefs_SetGet."Set", "error in (no error)"=w84, "VI Server Cluster"=w82) -> ("error out"=w83:errorcluster)  [unwired: 6 in, 2 out]
          }
          event "DI.Line", "DI.Port", "DI.Port.Lines.0:7", "DI.Port.Lines.8:15", "DI.Line.Update", "DI.Port.Update": Value Change {
            n153 = event-data() -> ("CtlRef"=w88:refnum<vi>)  [unwired: 1 in]
            n154 = call "NI_USB6212_Register_User_Last_Action.vi"("CtlRef"=w88, "error in (no error)"=w91, "VI Server Cluster"=w90) -> ("error out"=w89:errorcluster)  [unwired: 7 in, 1 out]
          }
          event "DO.Line.Update", "DO.Line", "DO.Port", "DO.Port.Lines.7:0", "DO.Port.Lines.15:8", "DO.Port.Update", "DO.Port.Lines.7:0.Mask", "DO.Port.Lines.15:8.Mask", "DO.Port.Mask.Apply": Value Change {
            n155 = event-data() -> ("CtlRef"=w92:refnum<vi>)  [unwired: 1 in]
            n156 = call "NI_USB6212_Register_User_Last_Action.vi"("CtlRef"=w92, "error in (no error)"=w95, "VI Server Cluster"=w93) -> ("error out"=w94:errorcluster)  [unwired: 7 in, 1 out]
          }
          event "Cntr.In.Channel", "Cntr.In.Input.Terminal", "Cntr.In.ActiveEdge", "Cntr.In.Sample.Clock.Source", "Cntr.In.IntegrationTime", "Cntr.In.Start": Value Change {
            n157 = event-data() -> ("CtlRef"=w96:refnum<vi>)  [unwired: 1 in]
            n158 = call "NI_USB6212_Register_User_Last_Action.vi"("CtlRef"=w96, "error in (no error)"=w99, "VI Server Cluster"=w97) -> ("error out"=w98:errorcluster)  [unwired: 7 in, 1 out]
          }
          event "Cntr.Out.Channel", "Cntr.Out.Output.Terminal", "Cntr.Out.Frequency", "Cntr.Out.Duty.Cycle", "Cntr.Out.Sample.Mode", "Cntr.Out.Start", "Cntr.Out.NumberOfPulces": Value Change {
            n159 = event-data() -> ("CtlRef"=w100:refnum<vi>)  [unwired: 1 in]
            n160 = call "NI_USB6212_Register_User_Last_Action.vi"("CtlRef"=w100, "error in (no error)"=w103, "VI Server Cluster"=w101) -> ("error out"=w102:errorcluster)  [unwired: 7 in, 1 out]
          }
        }
        n161 = call "Merge Errors II.vi"("error in 2 (no error)"=w32, "error in 1 (no error)"=w34) -> ("error out.DUP"=w33:errorcluster)  [unwired: 4 in, 1 out]
        n162 = call "NI_USB6212_Accessor_EXIT_Ref.vi"() -> ("EXIT"=w38:refnum<notifier>)  [unwired: 6 in]
        n163 = call "StopOnErrorOrCommand.vi"("STOP"=w38, "error in (no error)"=w33) -> ("error out"=w40:errorcluster, "STOP"=w39:bool)  [unwired: 8 in]
      }
      n164 = call "NI_USB6212_DAQmx_AI_Measure.vi"("error in (no error)"=w22, "VI Server Cluster"=w21) -> ("error out"=w20:errorcluster)  [unwired: 9 in]
      n165 = call "NI_USB6212_AO_Main_v2.vi"("error in (no error)"=w22, "VI Server Cluster"=w21) -> ("error out"=w24:errorcluster)  [unwired: 9 in]
      n166 = call "NI_USB6212_DAQmx_Counter_IN.vi"("error in (no error)"=w22, "VI Server Cluster"=w21) -> ("error out"=w26:errorcluster)  [unwired: 9 in]
      n167 = call "NI_USB6212_DAQmx_Counter_OUT.vi"("error in (no error)"=w22, "VI Server Cluster"=w21) -> ("error out"=w25:errorcluster)  [unwired: 9 in]
      n168 = call "NI_USB6212_Execute_Instructions_Processor.vi"("error in (no error)"=w22, "VI Server.RefsCluster"=w21) -> ("error out"=w23:errorcluster)  [unwired: 9 in]
      n169 = Build Array(w23, w25, w26, w24, w20, w30) -> (w27:errorcluster[])
      n170 = call "Merge Errors II.vi"("error array in"=w27, "error in 1 (no error)"=w29) -> ("error out.DUP"=w28:errorcluster)  [unwired: 4 in, 1 out]
    }
    frame Error {
    }
  }
  n171 = call-poly "VI Server_GetControl_Value_Ref.vi"("DataType"=tag "" ("DAQmx.Device"), "Control.Label"="DAQmx.Device", "error in"=w10, "SingleInstance"=TRUE, "VI Server.RefsCluster"=w7) -> ("error out"=w13:errorcluster, "Value"=w14:tag, "VI Server.RefsCluster.DUP"=w8:T3)  [unwired: 3 in, 1 out]
  n172 = call <vilib>:"DAQmx Reset Device.vi"("device in"=w14, "error in"=w13) -> ("error out"=w9:errorcluster)  [unwired: 13 in]
  n173 = call "VI Server_CloseRefs.vi"("error in"=w9, "VI Server.RefsCluster"=w8) -> ("error out"=w16:errorcluster)  [unwired: 9 in]
  n174 = call "NI_USB6212_Synch_CLOSE.vi"("error in"=w16) -> ("error out"=w5:errorcluster)  [unwired: 10 in]
  n175 = Current VI's Path() -> (path=w3:path)
  n176 = call "Close Window If in EXE mode.vi"("TopLevelVI Path"=w3, "error in"=w5) -> ("error out"=→"error out":errorcluster)  [unwired: 9 in]
